vi "Initialize.vi"(7 "HS (T) / LS (F)":bool=TRUE, 8 "error in (no error)":errorcluster) -> (0 "error out":errorcluster, 3 "TCP Writer out":refnum<class "TCP Writer.lvclass">)   [LabVIEW 2018, in "TCP Classes.lvlib" / "TCP Writer.lvclass"]
uses:
  TCP Writer.lvclass
  TCP Writer.lvclass/TCP Writer.ctl
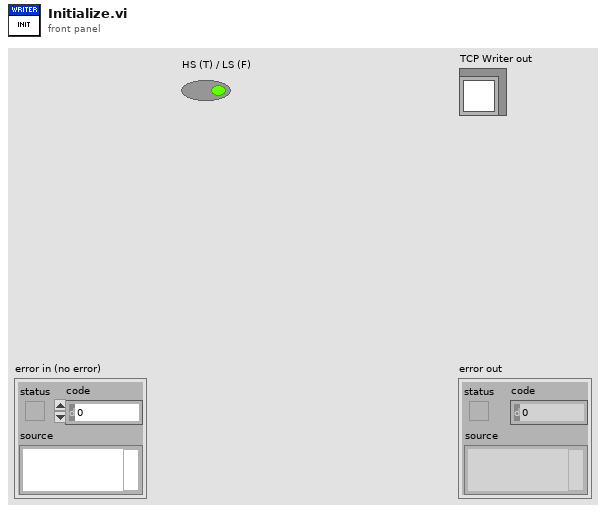
[diagram p1: front panel]
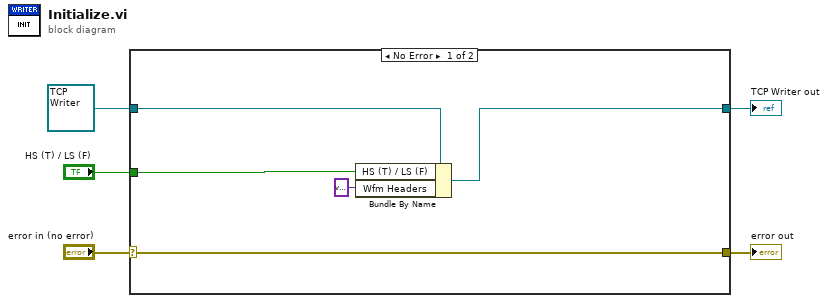
[diagram p0: block diagram]
diagram:
  n1 = case shown="No Error" "error in (no error)" {
    selector: "error in (no error)" -> [w7 w12]
    tunnel: [w7 w12] -> w4
    tunnel: [w8 w11] -> w2
    tunnel: refnum<class "TCP Writer.lvclass"> refnum ("TCP Writer in") -> [w10 w11]
    tunnel: "HS (T) / LS (F)" -> [w9 _]
    frame No Error {
      n2 = Bundle By Name(cluster=w10, "HS (T) / LS (F)"=w9, "Wfm Headers"=variant) -> (w8:refnum<class "TCP Writer.lvclass">)
    }
    frame Error {
    }
  }
  "error out" <- w4
  "TCP Writer out" <- w2
